vi "Spy Flush Errors.vi"(8 "error in (no error)":errorcluster, 11 "Mock Error Handler In":refnum<class "Mock Error Handler.lvclass">) -> (0 "error out":errorcluster, 1 "Errors":errorcluster[](array[cluster]), 2 "Locations":string[](array[string]), 3 "Mock Error Handler Out":refnum<class "Mock Error Handler.lvclass">)   [LabVIEW 2020, in "Mock Error Handler.lvclass"]
doc: "Spys on errors sent to the error handler. This Method requires a lock on the execution thread to prevent race conditions when testing other processes using the error handler."
uses:
  Mock Error Handler.lvclass
  Mock Error Handler.lvclass/Mock Error Handler.ctl
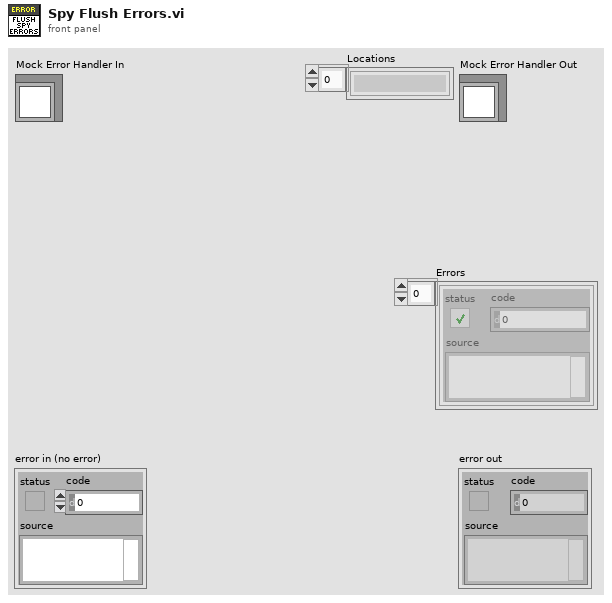
[diagram p1: front panel]
types:
  T1 = typedef "Mock Error Handler.lvclass/Error Message Data.ctl" = cluster{"Location":string, "Error":errorcluster}
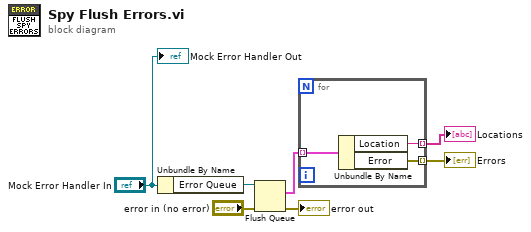
[diagram p0: block diagram]
diagram:
  n1 = Unbundle By Name("Mock Error Handler In") -> ("Error Queue"=w1:refnum<queue>)
  n2 = Flush Queue(queue=w1, error in (no error)="error in (no error)") -> (remaining elements=w2:T1[], error out=→"error out":errorcluster)  [unwired: 1 out]
  n3 = for {
    tunnel: w2 -> [w10] mode=indexing
    tunnel: [w9] -> w4 mode=indexing
    tunnel: [w8] -> w3 mode=indexing
    n4 = Unbundle By Name(w10) -> ("Location"=w9:string, "Error"=w8:errorcluster)
  }
  "Errors" <- w3
  "Locations" <- w4
  "Mock Error Handler Out" <- "Mock Error Handler In"
